vi "LCD_Custom_Command.vi"() -> ()   [LabVIEW 2020]
uses:
  <vilib>/MakerHub/LINX/Public/Utilities/Open Serial.vi
  <vilib>/MakerHub/LINX/LMH-LINX.lvlib
panel:
  out "Response":u8[](array[numeric])
  in  "stop":bool
  in  "Serial Port":refnum<visa-resource-name>="N/A"
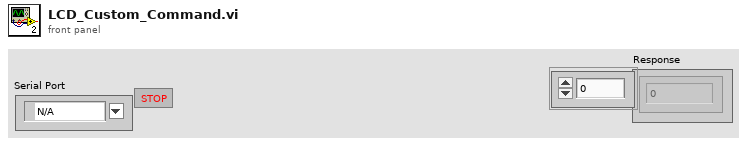
[diagram p1: front panel]
types:
  T1 = typedef "LMH-LINX.lvlib/LINX Ref.ctl" = cluster{"IO":T2, "Interface":T3, "LINX Device Config":T4}
  T2 = typedef "LMH-LINX.lvlib/Platform.ctl" = enum16{"Remote", "Local"}
  T3 = typedef "LMH-LINX.lvlib/Interface.ctl" = enum16{"Serial", "TCP"}
  T4 = typedef "LMH-LINX.lvlib/Device.lvlib/LINX Device Config.ctl" = cluster{"Interface":T3, "COM Port":refnum<visa-resource-name>, "TCP Configuration":T5, "Device Family":u8, "Device ID":u8, "Device Name":string, "TCP Ref":refnum<k5>, "Channels":T6}
  T5 = typedef "LMH-LINX.lvlib/Device.lvlib/TCP Config.ctl" = cluster{"IP Address":string, "Port":u16}
  T6 = typedef "LMH-LINX.lvlib/Channels.ctl" = cluster{"DI":u8[], "DO":u8[], "AI":u8[], "AO":u8[], "PWM":u8[], "QE":u8[], "UART":u8[], "I2C 2":u8[], "SPI":u8[], "CAN":u8[], "Servo":u8[], "AI Ref (V)":dbl, "AI Resolution (Bits)":u8, "AO Ref (V)":dbl, "AO Resolution (Bits)":u8}
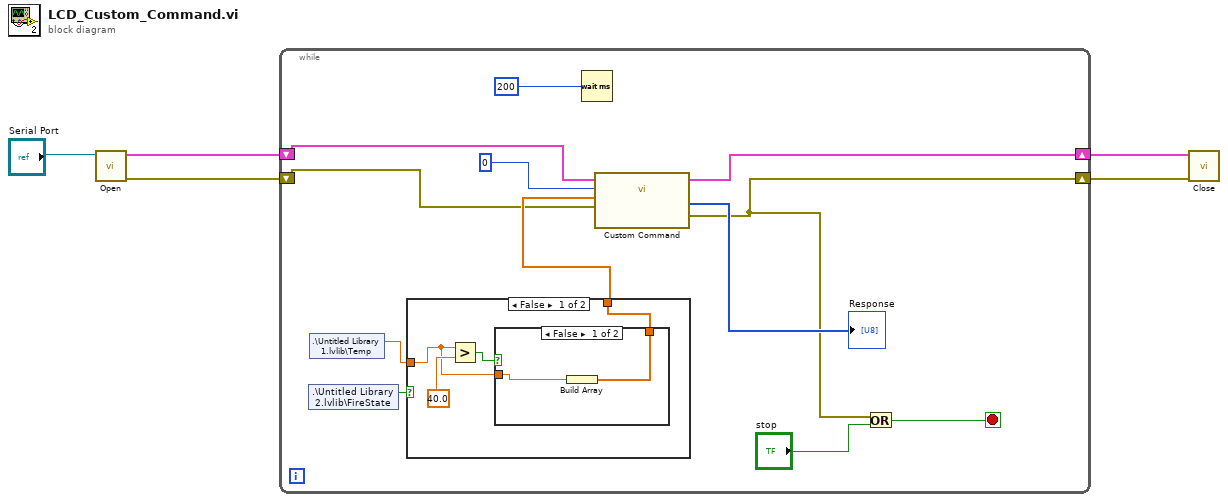
[diagram p0: block diagram]
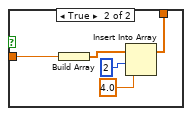
[diagram p2: hidden frame]
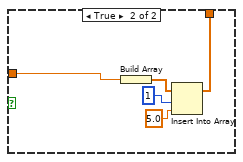
[diagram p3: hidden frame]
diagram:
  n1 = call-poly <vilib>:"Open.vi"("Serial Port"="Serial Port") -> ("Error Out"=w1:errorcluster, "LINX Resource"=w2:T1)  [unwired: 8 in, 1 out]
  n2 = while {
    shift-right: [w17] -> w5
    shift-left: w2 -> [w9]
    shift-right: [w13] -> w4
    shift-left: w1 -> [w8]
    stop <- w12 stop-if-true
    n3 = shared-variable ".\\Untitled Library 2.lvlib\\FireState"() -> (w6:bool)  [unwired: 1 in, 1 out]
    n4 = shared-variable ".\\Untitled Library 1.lvlib\\Temp"() -> (w7:dbl)  [unwired: 1 in, 1 out]
    n5 = case shown="False" w6 {
      tunnel: w7 -> [w19 w31]
      tunnel: [w18 w29] -> w10
      frame False {
        n6 = Greater?(x=w19, y=40.0) -> (0:w20:bool)
        n7 = case shown="False" w20 {
          tunnel: w19 -> [w23 w28]
          tunnel: [w22 w24] -> w18
          frame False {
            n8 = Build Array(w23) -> (w22:dbl[])
          }
          frame True {
            n9 = Build Array(w28) -> (w27:dbl[])
            n10 = Insert Into Array(array=w27, index=2, new element=4.0 ("new element/subarray")) -> (w24:dbl[])
          }
        }
      }
      frame True {
        n11 = Build Array(w31) -> (w30:dbl[])
        n12 = Insert Into Array(array=w30, index=1, new element=5.0 ("new element/subarray")) -> (w29:dbl[])
      }
    }
    n13 = Wait (ms)(milliseconds to wait=u32 200) -> ()  [unwired: 1 out]
    n14 = call <vilib>:"Custom Command.vi"("Error In"=w8, "Data"=w10, "Custom Command Number"=u16 0, "LINX Resource"=w9) -> ("Error Out"=w13:errorcluster, "Response"=→"Response":u8[], "LINX Resource"=w17:T1)  [unwired: 4 in, 1 out]
    n15 = Or(x=w13, y="stop") -> (x .or. y?=w12:bool)
  }
  n16 = call <vilib>:"Close.vi"("Error In"=w4, "LINX Resource"=w5) -> ()  [unwired: 9 in, 1 out]
